vi "isKingToKing.vi"(1 "Array":i32[][](array[numeric])) -> (0 "isKingToKing":bool)   [LabVIEW 2024]
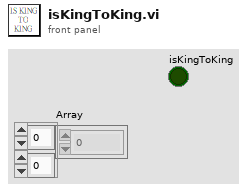
[diagram p1: front panel]
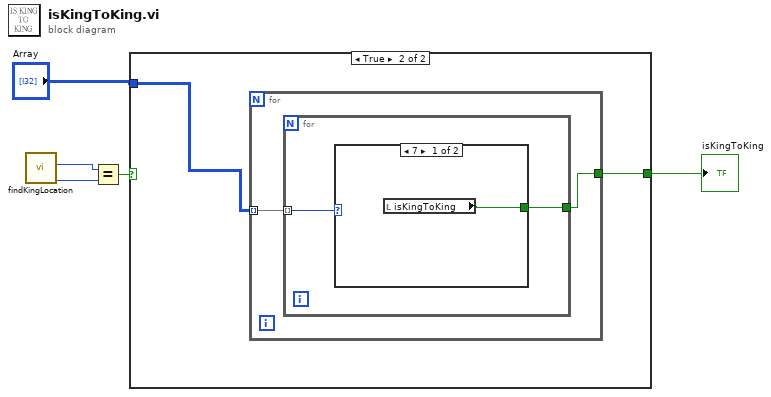
[diagram p0: block diagram]
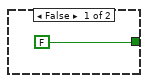
[diagram p2: hidden frame]
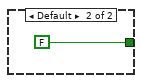
[diagram p3: hidden frame]
diagram:
  n1 = call "findKingLocation.vi"() -> ("bj"=w4:i32, "rj"=w3:i32)  [unwired: 2 out]
  n2 = Equal?(x=w3, y=w4) -> (x = y?=w5:bool)
  n3 = case shown="True" w5 {
    tunnel: [FALSE ("isKingToKing") w8] -> w2
    tunnel: "Array" -> [_ w7]
    frame False {
    }
    frame True {
      n4 = for {
        tunnel: w7 -> [w10] mode=indexing
        tunnel: [w9] -> w8
        n5 = for {
          tunnel: w10 -> [w12] mode=indexing
          tunnel: [w11] -> w9
          n6 = case shown="7" w12 {
            tunnel: [w13 FALSE ("isKingToKing")] -> w11
            frame 7 {
              n7 = local read "isKingToKing"() -> (w13:bool)
            }
            frame Default {
            }
          }
        }
      }
    }
  }
  "isKingToKing" <- w2
